vi "Write Pointer Size to Error.vi"(9 "offset":i32, 10 "Pointer":refnum<class "Pointer.lvclass">, 11 "error in":errorcluster) -> (1 "new offset":i32, 3 "error out":errorcluster)   [LabVIEW 2020, in "Memory Manager.lvlib" / "Pointer.lvclass"]
uses:
  Pointer.lvclass
  VIs/Write Numeric Scalar to Source (Base10 U64).vi
  Static Errors.lvlib
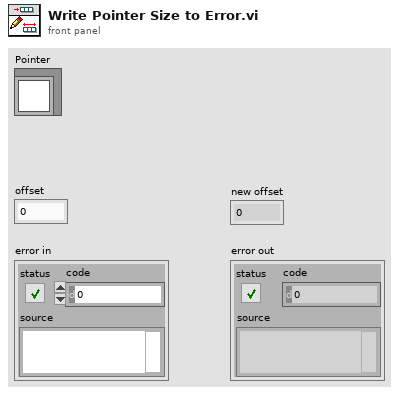
[diagram p1: front panel]
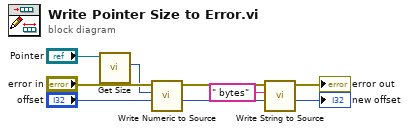
[diagram p0: block diagram]
diagram:
  n1 = call "Get Size.vi"("Pointer in"="Pointer") -> ("size"=w6:u64)  [unwired: 9 in, 1 out]
  n2 = call-poly "Write Numeric to Source.vi"("offset"="offset", "value"=w6, "error in"="error in") -> ("new offset"=w4:i32, "error out"=w5:errorcluster)  [unwired: 7 in]
  n3 = call "Write String to Source.vi"("offset"=w4, "string"=" bytes", "error in"=w5) -> ("new offset"=→"new offset":i32, "error out"=→"error out":errorcluster)  [unwired: 7 in]
